vi "Write Send Complete Service Msg.vi"(10 "Room Service Monitor UI.lvlib:Send Complete Service Msg.lvclass":refnum<class "Send Complete Service Msg.lvclass">, 11 "Room Service Monitor UI in":refnum<class "Room Service Monitor UI.lvclass">) -> (3 "Room Service Monitor UI out":refnum<class "Room Service Monitor UI.lvclass">)   [LabVIEW 2023, in "Room Service Monitor UI.lvlib" / "Room Service Monitor UI.lvclass"]
uses:
  Room Service Monitor UI.lvclass
  Room Service Monitor UI Messages/Send Complete Service Msg/Send Complete Service Msg.lvclass
  Room Service Monitor UI.lvclass/Room Service Monitor UI.ctl
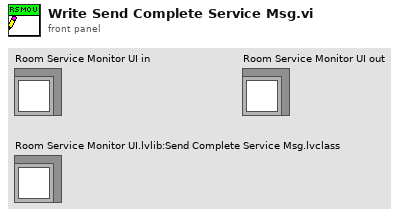
[diagram p1: front panel]
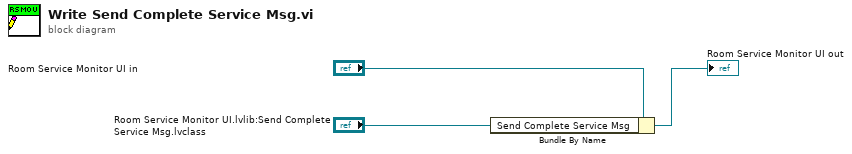
[diagram p0: block diagram]
diagram:
  n1 = Bundle By Name(cluster="Room Service Monitor UI in", "Send Complete Service Msg"="Room Service Monitor UI.lvlib:Send Complete Service Msg.lvclass") -> (→"Room Service Monitor UI out":refnum<class "Room Service Monitor UI.lvclass">)
